vi "CameraGuidage.vi"(0 "NumX in":i16=657, 1 "StartX":i16=1, 3 "Mode":u16(ring) items=["Exposition Guideur", "Calibration", "Guidage", "Piedestal", "Exposition simple", "Stop Guidage"], 4 "Duration":dbl=0.40000000000000013 min=0.0 step=0.1 format="%.2f", 5 "BinX":i16=1, 6 "NumberofImg":i32=1 caption="Nombre d'image" min=1 step=1, 7 "MaxIm.ICCDCamera":refnum<k7>, 9 "BinY":i16=1, 11 "NumY in":i16=495, 12 "StartY":i16=1, 14 "GuiderDeclination":i16) -> (8 "Done":bool, 10 "Error":errorcluster, 15 "GuiderArrayError":errorcluster)   [LabVIEW 2010]
uses:
  Globals.vi
panel:
  out "GuiderUpdate":bool=TRUE
  out "SaveImage":bool
  out "DarkImg":i32[][](array[numeric])
  in  "removedark":bool
  out "NumY dark":i16=495
  out "NumX dark":i16=657
  out "NumY out":i16=495
  out "NumX out":i16=657
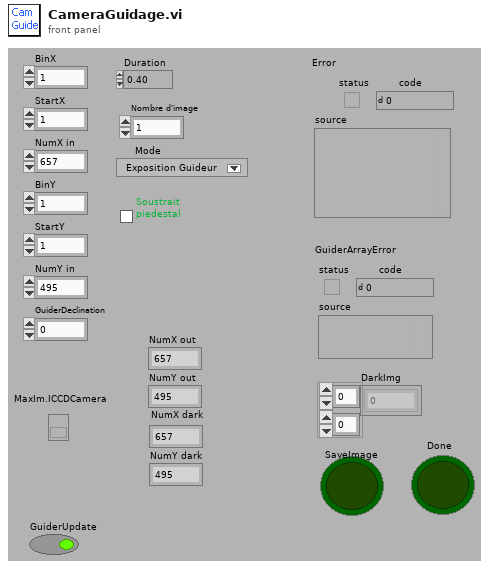
[diagram p1: front panel]
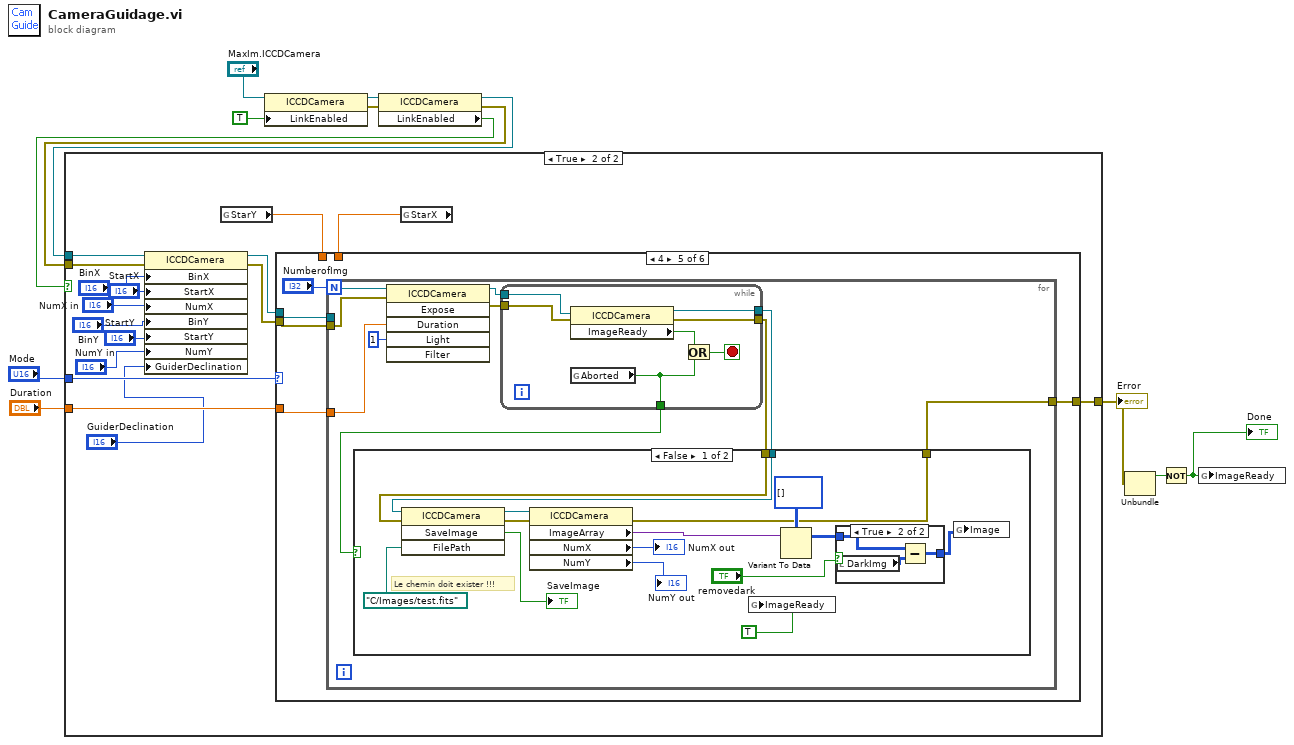
[diagram p0: block diagram]
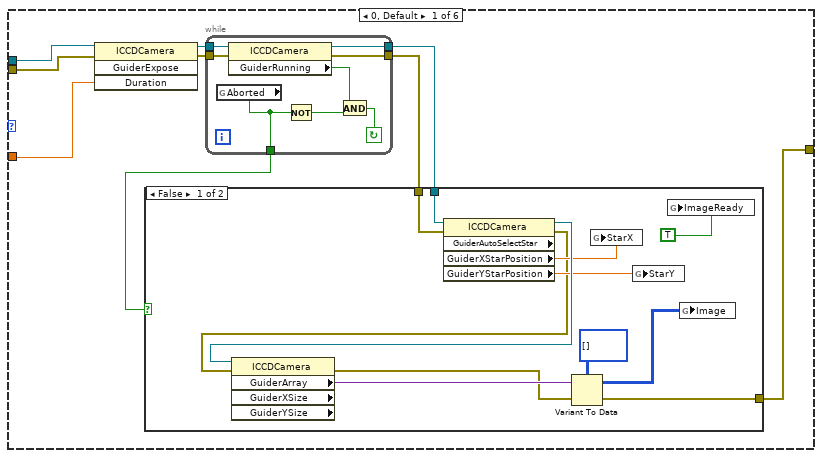
[diagram p3: hidden frame]
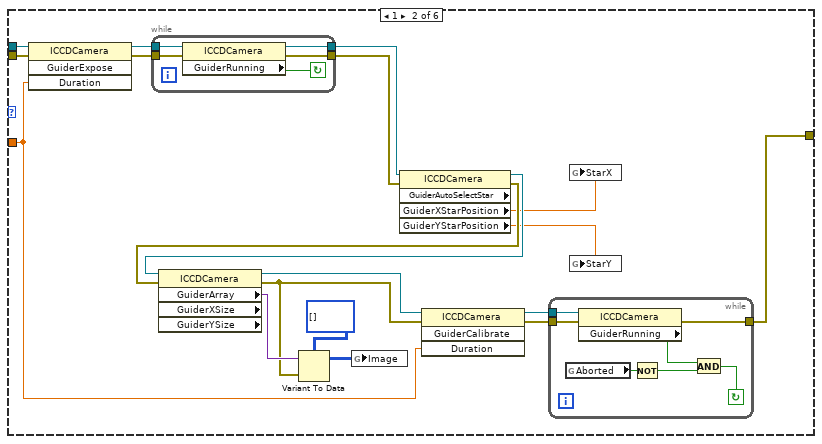
[diagram p5: hidden frame]
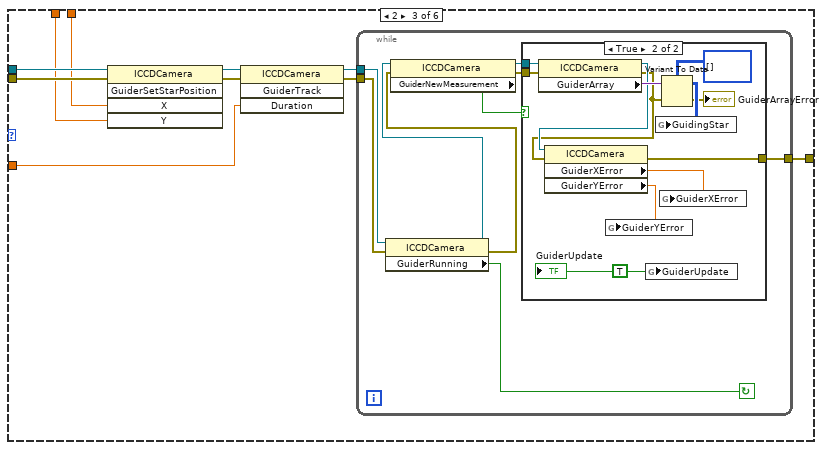
[diagram p6: hidden frame]
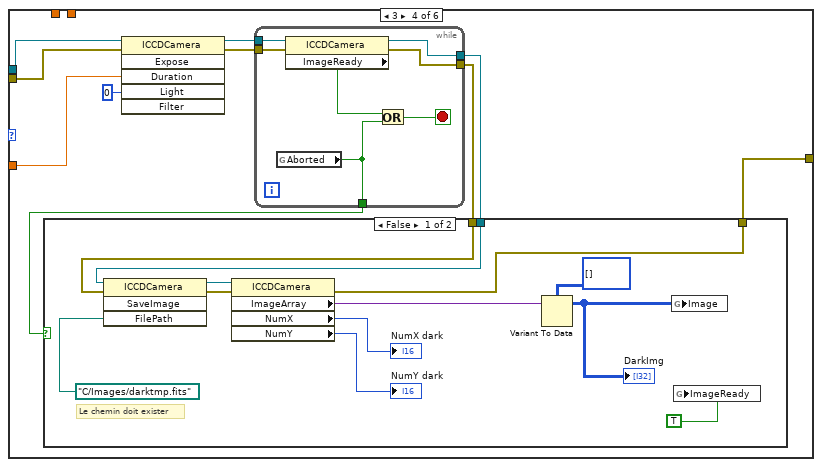
[diagram p8: hidden frame]
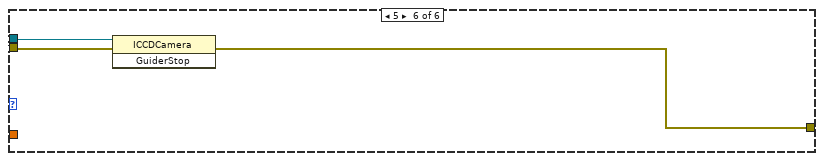
[diagram p12: hidden frame]
diagram:
  n1 = property class="ICCDCamera"(reference="MaxIm.ICCDCamera", "LinkEnabled"=TRUE) -> (reference out=w5:refnum<k7>, error out=w1:errorcluster)  [unwired: 1 in]
  n2 = property class="ICCDCamera"(reference=w5, error in=w1) -> (reference out=w10:refnum<k7>, error out=w9:errorcluster, "LinkEnabled"=w8:bool)
  n3 = case shown="True" w8 {
    tunnel: w10 -> [_ w27]
    tunnel: "Duration" -> [_ w29]
    tunnel: w9 -> [w13 w15]
    tunnel: [w13 w14] -> w6
    tunnel: "Mode" -> [_ w28]
    frame False {
    }
    frame True {
      n4 = property class="ICCDCamera"(reference=w27, error in=w15, "BinX"="BinX", "StartX"="StartX", "NumX"="NumX in", "BinY"="BinY", "StartY"="StartY", "NumY"="NumY in", "GuiderDeclination"="GuiderDeclination") -> (reference out=w26:refnum<k7>, error out=w25:errorcluster)
      n5 = global read "Globals.vi" "StarY"() -> (w16:sgl)
      n6 = global read "Globals.vi" "StarX"() -> (w17:sgl)
      n7 = case shown="4" w28 {
        tunnel: w26 -> [w35 w67 w99 w130 w157 w197]
        tunnel: w29 -> [w36 w63 w100 w127 w156 _]
        tunnel: w25 -> [w34 w66 w97 w126 w155 w196]
        tunnel: [w30 w76 w94 w124 w153 w195] -> w14
        tunnel: w17 -> [_ _ w92 _ _ _]
        tunnel: w16 -> [_ _ w93 _ _ _]
        frame 0, Default {
          n8 = invoke class="ICCDCamera" method="GuiderExpose"(reference=w35, error in=w34, "Duration"=w36) -> (reference out=w38:refnum<k7>, error out=w32:errorcluster)  [unwired: 1 in, 2 out]
          n9 = while {
            tunnel: [w56] -> w31
            tunnel: w32 -> [w57]
            tunnel: [w58] -> w37
            tunnel: w38 -> [w59]
            tunnel: [w52] -> w33
            stop <- w55 continue-if-true
            n10 = global read "Globals.vi" "Aborted"() -> (w52:bool)
            n11 = property class="ICCDCamera"(reference=w59, error in=w57) -> (reference out=w58:refnum<k7>, error out=w56:errorcluster, "GuiderRunning"=w54:bool)
            n12 = Not(x=w52) -> (.not. x?=w53:bool)
            n13 = And(x=w54, y=w53) -> (x .and. y?=w55:bool)
          }
          n14 = case shown="False" w33 {
            tunnel: w37 -> [w50 _]
            tunnel: w31 -> [w49 w51]
            tunnel: [w40 w51] -> w30
            frame False {
              n15 = property class="ICCDCamera" props=["GuiderAutoSelectStar", "GuiderXStarPosition", "GuiderYStarPosition"](reference=w50, error in=w49) -> (reference out=w48:refnum<k7>, error out=w39:errorcluster, "GuiderXStarPosition"=w44:sgl, "GuiderYStarPosition"=w43:sgl)  [unwired: 1 out]
              n16 = property class="ICCDCamera" props=["GuiderArray", "GuiderXSize", "GuiderYSize"](reference=w48, error in=w39) -> (error out=w41:errorcluster, "GuiderArray"=w47:variant)  [unwired: 3 out]
              n17 = Variant To Data(error in=w41, Variant=w47, type=i32[][] []) -> (error out=w40:errorcluster, data=w45:i32[][])
              n18 = global write "Globals.vi" "StarX"(w44) -> ()
              n19 = global write "Globals.vi" "StarY"(w43) -> ()
              n20 = global write "Globals.vi" "ImageReady"(TRUE) -> ()
              n21 = global write "Globals.vi" "Image"(w45) -> ()
            }
            frame True {
            }
          }
        }
        frame 1 {
          n22 = invoke class="ICCDCamera" method="GuiderExpose"(reference=w67, error in=w66, "Duration"=w63) -> (reference out=w75:refnum<k7>, error out=w74:errorcluster)  [unwired: 1 in, 2 out]
          n23 = while {
            tunnel: [w80] -> w72
            tunnel: w74 -> [w81]
            tunnel: [w82] -> w73
            tunnel: w75 -> [w83]
            stop <- w79 continue-if-true
            n24 = property class="ICCDCamera"(reference=w83, error in=w81) -> (reference out=w82:refnum<k7>, error out=w80:errorcluster, "GuiderRunning"=w79:bool)
          }
          n25 = property class="ICCDCamera" props=["GuiderAutoSelectStar", "GuiderXStarPosition", "GuiderYStarPosition"](reference=w73, error in=w72) -> (reference out=w71:refnum<k7>, error out=w70:errorcluster, "GuiderXStarPosition"=w60:sgl, "GuiderYStarPosition"=w61:sgl)  [unwired: 1 out]
          n26 = property class="ICCDCamera" props=["GuiderArray", "GuiderXSize", "GuiderYSize"](reference=w71, error in=w70) -> (reference out=w65:refnum<k7>, error out=w64:errorcluster, "GuiderArray"=w69:variant)  [unwired: 2 out]
          n27 = Variant To Data(error in=w64, Variant=w69, type=u32[][] []) -> (data=w62:u32[][])  [unwired: 1 out]
          n28 = global write "Globals.vi" "Image"(w62) -> ()
          n29 = invoke class="ICCDCamera" method="GuiderCalibrate"(reference=w65, error in=w64, "Duration"=w63) -> (reference out=w78:refnum<k7>, error out=w77:errorcluster)  [unwired: 1 in, 2 out]
          n30 = while {
            tunnel: [w88] -> w76
            tunnel: w77 -> [w89]
            tunnel: w78 -> [w90]
            stop <- w84 continue-if-true
            n31 = global read "Globals.vi" "Aborted"() -> (w87:bool)
            n32 = property class="ICCDCamera"(reference=w90, error in=w89) -> (error out=w88:errorcluster, "GuiderRunning"=w86:bool)  [unwired: 1 out]
            n33 = Not(x=w87) -> (.not. x?=w85:bool)
            n34 = And(x=w86, y=w85) -> (x .and. y?=w84:bool)
          }
          n35 = global write "Globals.vi" "StarX"(w60) -> ()
          n36 = global write "Globals.vi" "StarY"(w61) -> ()
        }
        frame 2 {
          n37 = invoke class="ICCDCamera" method="GuiderSetStarPosition"(reference=w99, error in=w97, "X"=w92, "Y"=w93) -> (reference out=w98:refnum<k7>, error out=w91:errorcluster)  [unwired: 1 in, 3 out]
          n38 = invoke class="ICCDCamera" method="GuiderTrack"(reference=w98, error in=w91, "Duration"=w100) -> (reference out=w96:refnum<k7>, error out=w95:errorcluster)  [unwired: 1 in, 2 out]
          n39 = while {
            tunnel: [w102] -> w94
            tunnel: w95 -> [w105]
            tunnel: w96 -> [w106]
            stop <- w101 continue-if-true
            n40 = property class="ICCDCamera"(reference=w106, error in=w105) -> (reference out=w103:refnum<k7>, error out=w104:errorcluster, "GuiderRunning"=w101:bool)
            n41 = property class="ICCDCamera"(reference=w103, error in=w104) -> (reference out=w107:refnum<k7>, error out=w108:errorcluster, "GuiderNewMeasurement"=w109:bool)
            n42 = case shown="True" w109 {
              tunnel: w108 -> [w110 w112]
              tunnel: [w110 w120] -> w102
              tunnel: w107 -> [_ w119]
              frame False {
              }
              frame True {
                w111 = TRUE ("GuiderUpdate")
                n43 = property class="ICCDCamera"(reference=w119, error in=w112) -> (reference out=w115:refnum<k7>, error out=w113:errorcluster, "GuiderArray"=w118:variant)
                n44 = property class="ICCDCamera"(reference=w115, error in=w113) -> (error out=w120:errorcluster, "GuiderXError"=w122:sgl, "GuiderYError"=w121:sgl)  [unwired: 1 out]
                n45 = global write "Globals.vi" "GuiderYError"(w121) -> ()
                n46 = global write "Globals.vi" "GuiderUpdate"(w111) -> ()
                n47 = global write "Globals.vi" "GuiderXError"(w122) -> ()
                n48 = Variant To Data(error in=w113, Variant=w118, type=u32[][] []) -> (error out=→"GuiderArrayError":errorcluster, data=w117:u32[][])
                n49 = global write "Globals.vi" "GuidingStar"(w117) -> ()
                "GuiderUpdate" <- w111
              }
            }
          }
        }
        frame 3 {
          n50 = invoke class="ICCDCamera" method="Expose"(reference=w130, error in=w126, "Duration"=w127, "Light"=i16 0) -> (reference out=w132:refnum<k7>, error out=w129:errorcluster)  [unwired: 2 in, 4 out]
          n51 = while {
            tunnel: [w149] -> w128
            tunnel: w129 -> [w150]
            tunnel: [w151] -> w131
            tunnel: w132 -> [w152]
            tunnel: [w146] -> w123
            stop <- w148 stop-if-true
            n52 = global read "Globals.vi" "Aborted"() -> (w146:bool)
            n53 = property class="ICCDCamera"(reference=w152, error in=w150) -> (reference out=w151:refnum<k7>, error out=w149:errorcluster, "ImageReady"=w147:bool)
            n54 = Or(x=w147, y=w146) -> (x .or. y?=w148:bool)
          }
          n55 = case shown="False" w123 {
            tunnel: w131 -> [w144 _]
            tunnel: w128 -> [w143 w145]
            tunnel: [w136 w145] -> w124
            frame False {
              # "Le chemin doit exister"
              n56 = invoke class="ICCDCamera" method="SaveImage"(reference=w144, error in=w143, "FilePath"=path "C:/Images/darktmp.fits") -> (reference out=w142:refnum<k7>, error out=w139:errorcluster)  [unwired: 1 in, 2 out]
              n57 = property class="ICCDCamera"(reference=w142, error in=w139) -> (error out=w136:errorcluster, "ImageArray"=w141:variant, "NumX"=→"NumX dark":i16, "NumY"=→"NumY dark":i16)  [unwired: 1 out]
              n58 = Variant To Data(Variant=w141, type=i32[][] []) -> (data=w134:i32[][])  [unwired: 1 in, 1 out]
              "DarkImg" <- w134
              n59 = global write "Globals.vi" "Image"(w134) -> ()
              n60 = global write "Globals.vi" "ImageReady"(TRUE) -> ()
            }
            frame True {
            }
          }
        }
        frame 4 {
          n61 = for {
            N: "NumberofImg" -> [_]
            tunnel: w157 -> [w165]
            tunnel: w156 -> [w162]
            tunnel: [w161] -> w153
            tunnel: w155 -> [w160]
            n62 = invoke class="ICCDCamera" method="Expose"(reference=w165, error in=w160, "Duration"=w162, "Light"=i16 1) -> (reference out=w167:refnum<k7>, error out=w164:errorcluster)  [unwired: 2 in, 4 out]
            n63 = while {
              tunnel: [w191] -> w163
              tunnel: w164 -> [w192]
              tunnel: [w193] -> w166
              tunnel: w167 -> [w194]
              tunnel: [w188] -> w158
              stop <- w190 stop-if-true
              n64 = property class="ICCDCamera"(reference=w194, error in=w192) -> (reference out=w193:refnum<k7>, error out=w191:errorcluster, "ImageReady"=w189:bool)
              n65 = global read "Globals.vi" "Aborted"() -> (w188:bool)
              n66 = Or(x=w189, y=w188) -> (x .or. y?=w190:bool)
            }
            n67 = case shown="False" w158 {
              tunnel: w166 -> [w182 _]
              tunnel: w163 -> [w181 w187]
              tunnel: [w174 w187] -> w161
              frame False {
                # "Le chemin doit exister !!!"
                n68 = invoke class="ICCDCamera" method="SaveImage"(reference=w182, error in=w181, "FilePath"=path "C:/Images/test.fits") -> (reference out=w180:refnum<k7>, error out=w175:errorcluster, "SaveImage"=→"SaveImage":bool)  [unwired: 1 in, 1 out]
                n69 = property class="ICCDCamera"(reference=w180, error in=w175) -> (error out=w174:errorcluster, "ImageArray"=w179:variant, "NumX"=→"NumX out":i16, "NumY"=→"NumY out":i16)  [unwired: 1 out]
                n70 = global write "Globals.vi" "ImageReady"(TRUE) -> ()
                n71 = Variant To Data(Variant=w179, type=i32[][] []) -> (data=w171:i32[][])  [unwired: 1 in, 1 out]
                n72 = case shown="True" "removedark" {
                  tunnel: w171 -> [w183 w186]
                  tunnel: [w183 w184] -> w170
                  frame False {
                  }
                  frame True {
                    n73 = local read "DarkImg"() -> (w185:i32[][])
                    n74 = Subtract(x=w186, y=w185) -> (x-y=w184:i32[][])
                  }
                }
                n75 = global write "Globals.vi" "Image"(w170) -> ()
              }
              frame True {
              }
            }
          }
        }
        frame 5 {
          n76 = invoke class="ICCDCamera" method="GuiderStop"(reference=w197, error in=w196) -> (error out=w195:errorcluster)  [unwired: 1 in, 2 out]
        }
      }
    }
  }
  "Error" <- w6
  n77 = Unbundle(w6) -> ("status"=w4:bool)  [unwired: 2 out]
  n78 = Not(x=w4) -> (.not. x?=w2:bool)
  "Done" <- w2
  n79 = global write "Globals.vi" "ImageReady"(w2) -> ()
